vi "set_control_in_Memory.vi"(3 "Control Name":string, 4 "Value":variant, 5 "VI Name":string="Client with Signaling") -> (0 "error out 2":errorcluster)   [LabVIEW 2020]
panel:
  in  "vi reference":refnum<vi>
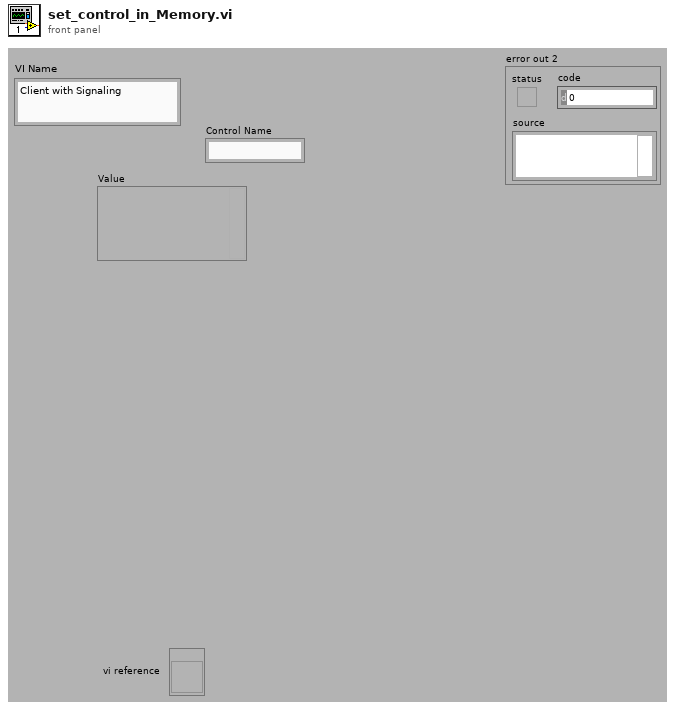
[diagram p1: front panel]
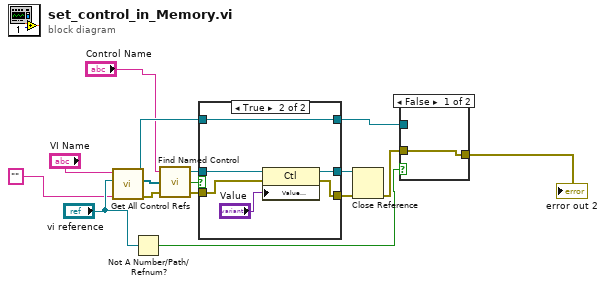
[diagram p0: block diagram]
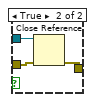
[diagram p2: hidden frame]
diagram:
  n1 = call "Get All Control Refs.vi"("VI Name"="VI Name", "vi reference"="vi reference", "Machine Name"="") -> ("VI Refnum"=w8:refnum<vi>, "All Controls"=w14:refnum<vi>[], "error out"=w13:errorcluster)  [unwired: 3 in]
  n2 = Not A Number/Path/Refnum?(number/path/refnum="vi reference") -> (NaN/Path/Refnum?=w5:bool)
  n3 = call "Find Named Control.vi"("error in"=w13, "All Controls"=w14, "Control Name"="Control Name") -> ("error out"=w10:errorcluster, "Found"=w11:bool, "Ctl Refnum"=w12:refnum<vi>)
  n4 = case shown="True" w11 {
    tunnel: w12 -> [w18 w25]
    tunnel: [w18 w24] -> w16
    tunnel: [w19 w23] -> w15
    tunnel: w10 -> [w19 w22]
    tunnel: w8 -> [w17 w21]
    tunnel: [w17 w21] -> w9
    frame False {
    }
    frame True {
      n5 = property class="Ctl"(reference=w25, error in=w22, "Value (Signaling)"="Value") -> (reference out=w24:refnum<vi>, error out=w23:errorcluster)
    }
  }
  n6 = Close Reference(reference=w16, error in (no error)=w15) -> (error out=w7:errorcluster)
  n7 = case shown="False" w5 {
    tunnel: w9 -> [_ w29]
    tunnel: w7 -> [w26 w28]
    tunnel: [w26 w27] -> w2
    frame False {
    }
    frame True {
      n8 = Close Reference(reference=w29, error in (no error)=w28) -> (error out=w27:errorcluster)
    }
  }
  "error out 2" <- w2
